vi "Day 13.1 - First Fold.vi"(11 "input":string) -> (3 "output":i32)   [LabVIEW 2021]
panel:
  out "output array":bool[][](array[boolean])
  out "original array":bool[][](array[boolean])
  out "number":string[](array[string])
  out "Fold":string[](array[string])
  out "dots":i32[][](array[numeric])
  out "Folds":string
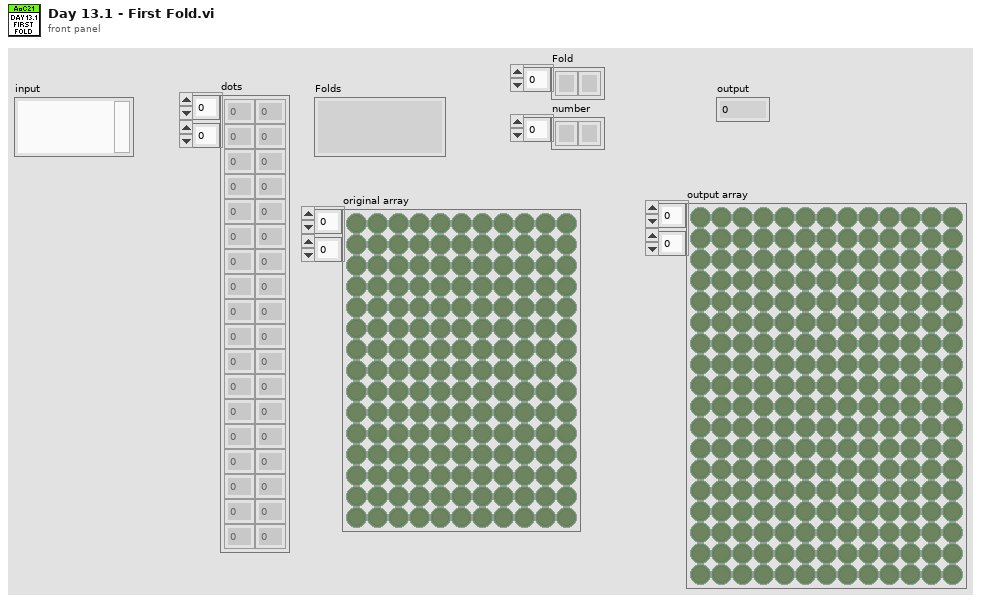
[diagram p1: front panel]
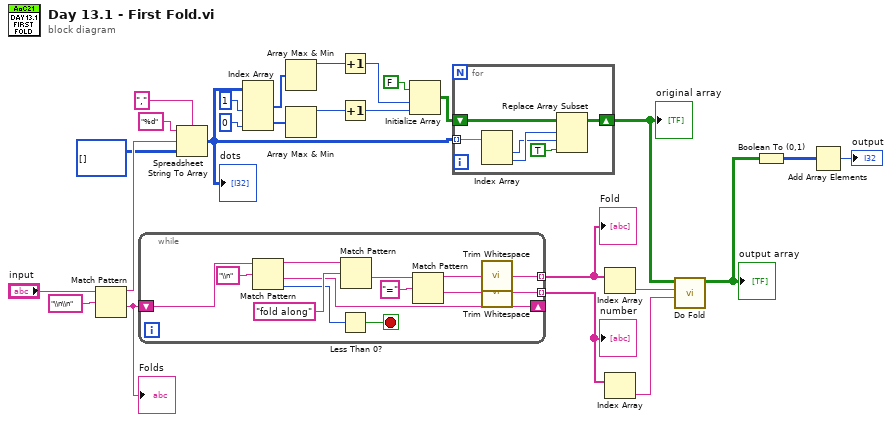
[diagram p0: block diagram]
diagram:
  n1 = Match Pattern(string="input", regular expression="\\n\\n") -> (before substring=w24:string, after substring=w3:string)  [unwired: 1 in, 2 out]
  "Folds" <- w3
  n2 = while {
    tunnel: [w33] -> w2 mode=indexing
    tunnel: [w32] -> w1 mode=indexing
    shift-right: [w28] -> _
    shift-left: w3 -> [w30]
    stop <- w36 stop-if-true
    n3 = Match Pattern(string=w30, regular expression="\\n") -> (before substring=w29:string, after substring=w28:string, offset past match=w27:i32)  [unwired: 1 in, 1 out]
    n4 = Less Than 0?(x=w27) -> (x < 0?=w36:bool)
    n5 = Match Pattern(string=w29, regular expression="fold along") -> (after substring=w38:string)  [unwired: 1 in, 3 out]
    n6 = Match Pattern(string=w38, regular expression="=") -> (before substring=w35:string, after substring=w34:string)  [unwired: 1 in, 2 out]
    n7 = call <vilib>:"Trim Whitespace.vi"("string"=w35) -> ("trimmed string"=w33:string)  [unwired: 1 in]
    n8 = call <vilib>:"Trim Whitespace.vi"("string"=w34) -> ("trimmed string"=w32:string)  [unwired: 1 in]
  }
  "Fold" <- w2
  "number" <- w1
  n9 = Spreadsheet String To Array(delimiter (Tab)=",", format string="%d", spreadsheet string=w24, array type (2D Dbl)=i32[][] []) -> (array=w13:i32[][])
  "dots" <- w13
  n10 = Index Array(array=w13, index (col) #1=1 ("disabled index (col)"), index (col) #2=0 ("index (col)")) -> (element #1=w15:i32[], element #2=w16:i32[])  [unwired: 2 in]
  n11 = Array Max & Min(array=w15) -> (max value=w14:i32)  [unwired: 3 out]
  n12 = Array Max & Min(array=w16) -> (max value=w17:i32)  [unwired: 3 out]
  n13 = Increment(x=w14) -> (x+1=w11:i32)
  n14 = Increment(x=w17) -> (x+1=w10:i32)
  n15 = Initialize Array(FALSE, w11, w10) -> (w12:bool[][])
  n16 = for {
    tunnel: w13 -> [w43] mode=indexing
    shift-right: [w44] -> w7
    shift-left: w12 -> [w45]
    n17 = Index Array(array=w43) -> (element #1=w40:i32, element #2=w41:i32)  [unwired: 2 in]
    n18 = Replace Array Subset(array=w45, new element=TRUE ("new element/subarray"), index (row)=w41, index (col)=w40) -> (w44:bool[][])
  }
  "original array" <- w7
  n19 = Index Array(array=w2) -> (element=w9:string)  [unwired: 1 in]
  n20 = Index Array(array=w1) -> (element=w8:string)  [unwired: 1 in]
  n21 = call "Do Fold.vi"("Fold Line"=w8, "Fold Axis"=w9, "Array in"=w7) -> ("Array out"=w6:bool[][])  [unwired: 8 in]
  "output array" <- w6
  n22 = Boolean To (0,1)(Boolean=w6) -> (0, 1=w5:i16[][])
  n23 = Add Array Elements(numeric array=w5) -> (sum=→"output":i16)
